vi "Quadratic Programming.vi"   [LabVIEW 2012, in "NI_Gmath.lvlib"]
doc: "Uses either an interior point algorithm or an active set algorithm to solve the problem: minimize 0.5x*Q*x + c*x, such that A*x=b and <B>Imin</B> are less than or equal to D*x, which is less than or equal to <B>Imax</B>. You must manually select the polymorphic instance to use."
uses:
  NI_Gmath.lvlib
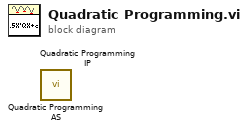
[diagram p0: block diagram]
diagram:
  n1 = call "Quadratic Programming AS.vi"() -> ()  [unwired: 8 in, 4 out]
  n2 = call "Quadratic Programming IP.vi"() -> ()  [unwired: 8 in, 4 out]
